vi "Get Hardware Version.vi"(0 "PCB":u32, 1 "CameraFirmwareVersion":u32, 5 "Decode":u32, 7 "dummy1":u32, 9 "dummy2":u32, 12 "CameraFirmwareBuild":u32) -> (2 "function return":u32, 3 "CameraFirmwareVersion out":u32, 4 "PCB out":u32, 6 "Decode out":u32, 8 "dummy1 out":u32, 10 "dummy2 out":u32, 14 "CameraFirmwareBuild out":u32)   [LabVIEW 2018, in "AndorSDK.lvlib"]
doc: "EXPNETTYPE unsigned int WINAPI GetHardwareVersion(unsigned int * PCB, unsigned int * Decode, unsigned int * dummy1, unsigned int * dummy2, unsigned int * CameraFirmwareVersion, unsigned int * CameraFirmwareBuild);"
uses:
  AndorSDK.lvlib
  ATMCD32D.dll
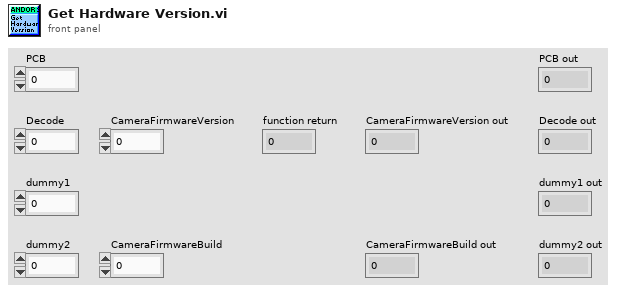
[diagram p1: front panel]
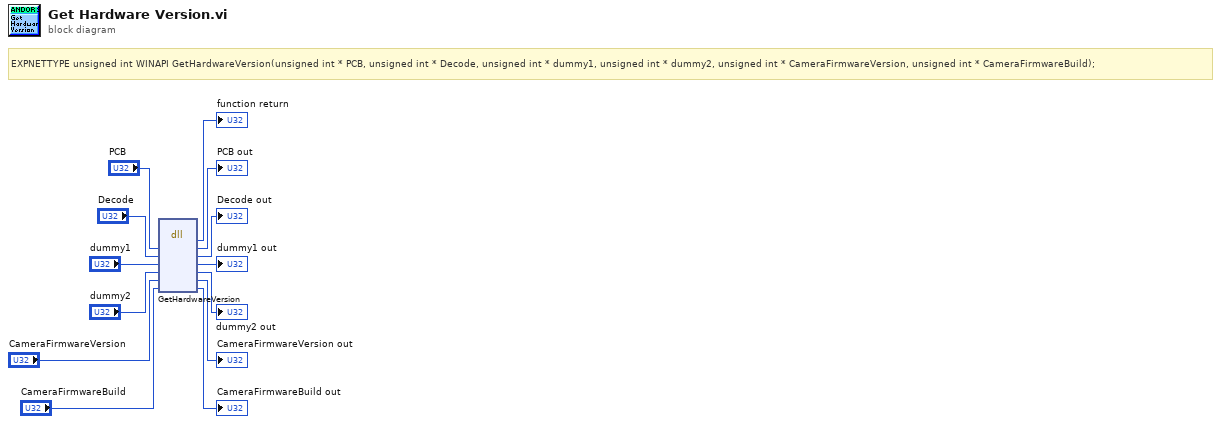
[diagram p0: block diagram]
diagram:
  # "EXPNETTYPE unsigned int WINAPI GetHardwareVersion(unsigned int * PCB, unsigned int * Decode, unsigned int * dummy1, unsigned int * dummy2, unsigned int * CameraFirmwareVersion, unsigned int * CameraFirmwareBuild);"
  n1 = dll-call lib="PTH2babs E\nPersönliches02 - Arbeit03-HiwijobsLabviewCodelibANDOR\tAndor SDK\nATMCD32D.*" fn="GetHardwareVersion"("PCB"="PCB", "Decode"="Decode", "dummy1"="dummy1", "dummy2"="dummy2", "CameraFirmwareVersion"="CameraFirmwareVersion", "CameraFirmwareBuild"="CameraFirmwareBuild") -> (→"function return":u32, "PCB"=→"PCB out":u32, "Decode"=→"Decode out":u32, "dummy1"=→"dummy1 out":u32, "dummy2"=→"dummy2 out":u32, "CameraFirmwareVersion"=→"CameraFirmwareVersion out":u32, "CameraFirmwareBuild"=→"CameraFirmwareBuild out":u32)  [unwired: 3 in, 2 out]
